vi "acquire_FXP_18-5_FIFO_1.vi"(6 "numChannels":u32, 7 "Iters":i32, 8 "error in":errorcluster, 11 "FPGA Interface":T1) -> (0 "error out":errorcluster, 1 "Elements Remaining":u32, 2 "2D Data Out":dbl[][](array[numeric]), 3 "acquisition done":bool, 5 "u iter":i32)   [LabVIEW 2017, in "fpga_interface.lvlib"]
uses:
  fpga_interface.lvlib
  <vilib>/rvi/interface/nirviMethod/nirviMethod.xnode
  <vilib>/FPGAPlugInAG/Dynamic/niLvFpga_ReadFifo_Dynamic.vi
  <vilib>/rvi/errors/niLvFpgaMergeErrorWithErrorCode.vi
  fpga_interface_types/FPGA_to_HOST_1_FXP_18-5_FIFO_interface.ctl
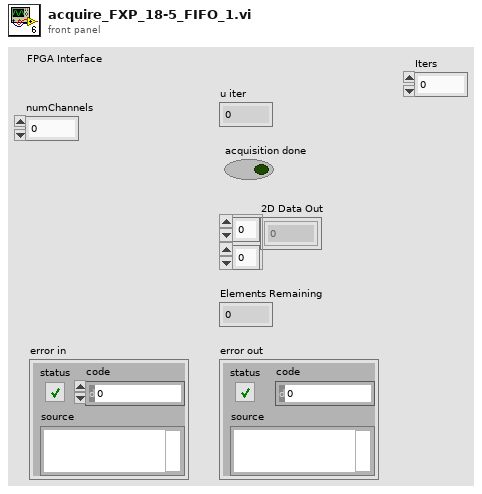
[diagram p1: front panel]
types:
  T1 = typedef "fpga_interface.lvlib/FPGA_to_HOST_1_FXP_18-5_FIFO_interface.ctl" = refnum<k20>
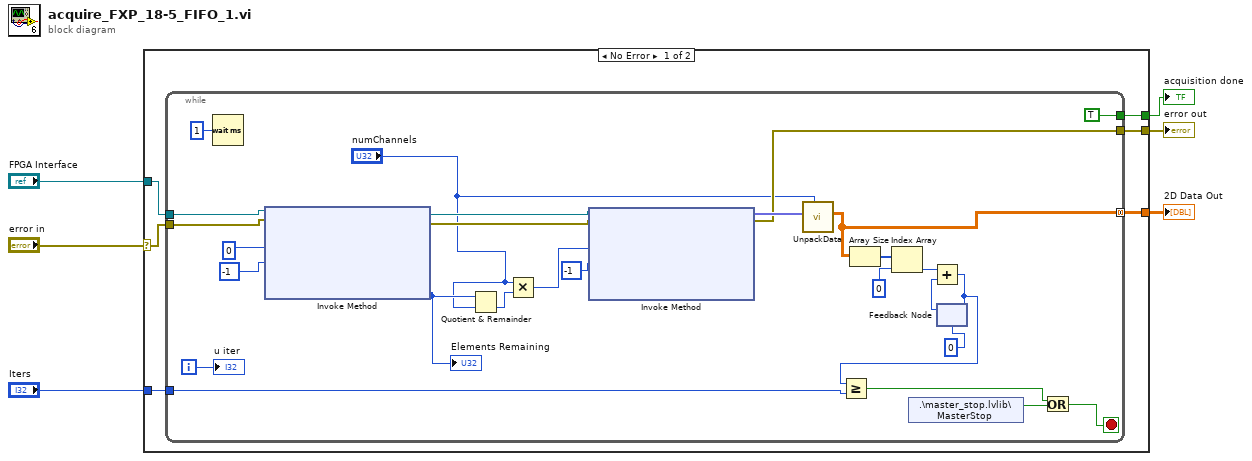
[diagram p0: block diagram]
diagram:
  n1 = case shown="No Error" "error in" {
    selector: "error in" -> [w7 w40]
    tunnel: [w12 _] -> w6
    tunnel: [w11 w40] -> w5
    tunnel: [w10 _] -> w4
    tunnel: "Iters" -> [w9 _]
    tunnel: "FPGA Interface" -> [w8 _]
    frame No Error {
      n2 = while {
        tunnel: [w34] -> w10 mode=concatenating
        tunnel: w8 -> [w28]
        tunnel: w7 -> [w27]
        tunnel: [w25] -> w11
        tunnel: [TRUE] -> w12
        tunnel: w9 -> [w16]
        i -> [w36]
        stop <- w21 stop-if-true
        n3 = Wait (ms)(milliseconds to wait=u32 1) -> ()  [unwired: 1 out]
        n4 = xnode "Invoke Method"("FPGA VI Reference In"=w28, "error in"=w27, "Number of Elements"=0 ("Timeout (ms)"), "Timeout (ms)"=-1) -> ("FPGA VI Reference Out"=w22:T1, "error out"=w24:errorcluster, "Elements Remaining"=w31:u32)  [unwired: 1 out]
        "Elements Remaining" <- w31
        n5 = Quotient & Remainder(x=w31, y="numChannels") -> (floor(x/y)=w38:u32)  [unwired: 1 out]
        n6 = Multiply(x="numChannels", y=w38) -> (x*y=w13:u32)
        n7 = xnode "Invoke Method"("FPGA VI Reference In"=w22, "error in"=w24, "Number of Elements"=w13, "Timeout (ms)"=-1) -> ("error out"=w25:errorcluster, "Data"=w26:fxp<+/-,18,5>[])  [unwired: 2 out]
        n8 = call "UnpackData.vi"("NumChannels"="numChannels", "1D Data In"=w26) -> ("2D Data Out"=w34:dbl[][])  [unwired: 8 in, 1 out]
        n9 = Array Size(array=w34) -> (size(s)=w32:i32[])
        n10 = Index Array(array=w32, index=0) -> (element=w35:i32)
        n11 = shared-variable ".\\master_stop.lvlib\\MasterStop"() -> (w19:bool)  [unwired: 1 in, 1 out]
        n12 = feedback #1(0) -> (w37:i32)
        n13 = Add(x=w35, y=w37) -> (x+y=w17:i32)
        n14 = Greater Or Equal?(x=w17, y=w16) -> (x >= y?=w20:bool)
        n15 = feedback-in #1(w17) -> ()
        n16 = Or(x=w20, y=w19) -> (x .or. y?=w21:bool)
        "u iter" <- w36
      }
    }
    frame Error {
    }
  }
  "acquisition done" <- w6
  "error out" <- w5
  "2D Data Out" <- w4
